vi "Categorize Terminals and Names.vi"(10 "terminal names":string[](array[string]), 11 "terminal addresses":T1[](array[typedef])) -> (1 "map from terminal address (string) to terminal name":map{string, string}(c390), 2 "remote terminals":string[](array[string]), 3 "bus controller":string[](array[string]))   [LabVIEW 2020, in "AIM MIL-STD-1553 System Explorer.lvlib" / "Implementation.lvlib" / "Refresh.lvlib"]
uses:
  Refresh.lvlib
  Scripting/AIM MIL-STD-1553 Scripting.lvlib
  Shared/Address.ctl
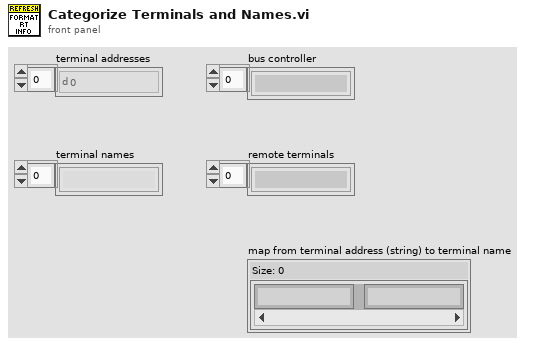
[diagram p1: front panel]
types:
  T1 = typedef "Address.ctl" = u16
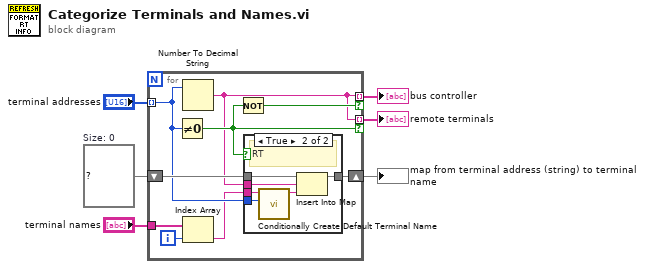
[diagram p0: block diagram]
diagram:
  w5 = map{string, string} {}  # Size: 0
  n1 = for {
    tunnel: "terminal addresses" -> [w8] mode=indexing
    tunnel: [w9] -> w1 mode=indexing if=w13
    tunnel: [w9] -> w4 mode=indexing if=w12
    tunnel: "terminal names" -> [w15]
    shift-right: [w10] -> w6
    shift-left: w5 -> [w11]
    i -> [w14]
    n2 = Not Equal To 0?(x=w8) -> (x != 0?=w12:bool)
    n3 = Number To Decimal String(number=w8) -> (decimal integer string=w9:string)  [unwired: 1 in]
    n4 = Index Array(array=w15, index=w14) -> (element=w7:string)
    n5 = Not(x=w12) -> (.not. x?=w13:bool)
    n6 = case shown="True" w12 {
      tunnel: w11 -> [w16 w22]
      tunnel: [w16 w20] -> w10
      tunnel: w9 -> [_ w21]
      tunnel: w8 -> [_ w19]
      tunnel: w7 -> [_ w18]
      frame False {
        # "BC"
      }
      frame True {
        # "RT"
        n7 = call "Conditionally Create Default Terminal Name.vi"("terminal address in"=w19, "terminal name in"=w18) -> ("terminal name out"=w17:string)  [unwired: 8 in, 1 out]
        n8 = Insert Into Map(map in=w22, key=w21, value=w17) -> (map out=w20:map{string, string})  [unwired: 2 out]
      }
    }
  }
  "map from terminal address (string) to terminal name" <- w6
  "remote terminals" <- w4
  "bus controller" <- w1
